vi "Merge Results.vi"(8 "error in (no error)":errorcluster, 9 "Merge in  front":bool, 10 "Result in":refnum<class "Acquired Result.lvclass">, 11 "Response Synchronizer in":refnum<class "Response Synchronizer.lvclass">) -> (0 "error out":errorcluster, 2 "Merged Result":refnum<class "Acquired Result.lvclass">, 3 "Response Synchronizer out":refnum<class "Response Synchronizer.lvclass">)   [LabVIEW 2021, in "Response Synchronizer.lvclass"]
uses:
  Response Synchronizer.lvclass
  NHMFL_Core/Libraries/Instruments/Results/Acquired Result/Acquired Result.lvclass
  Response Synchronizer.lvclass/Response Synchronizer.ctl
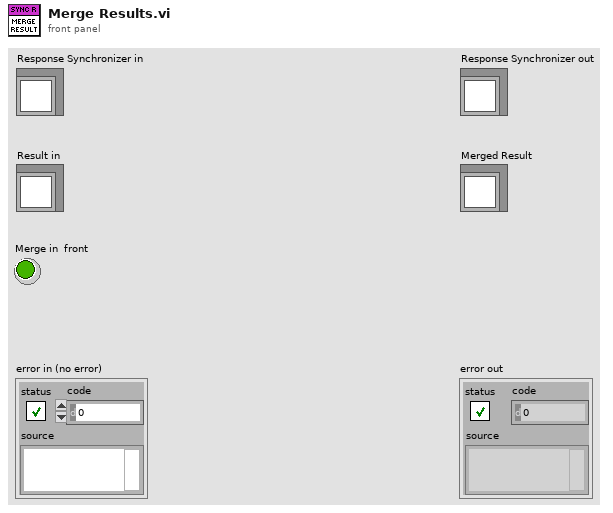
[diagram p1: front panel]
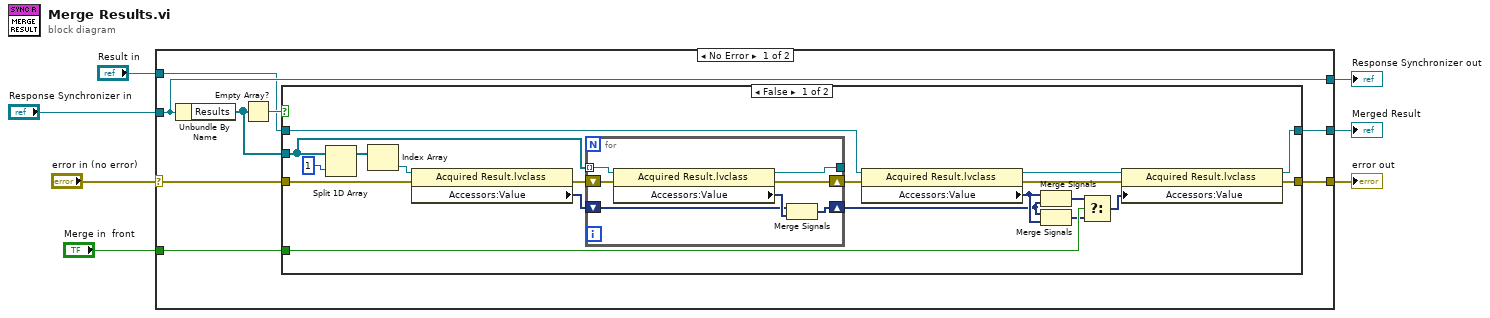
[diagram p0: block diagram]
diagram:
  n1 = case shown="No Error" "error in (no error)" {
    selector: "error in (no error)" -> [w9 w46]
    tunnel: [w8 w46] -> w6
    tunnel: [w15 w45] -> w4
    tunnel: "Response Synchronizer in" -> [w15 w45]
    tunnel: [w12 w44] -> w3
    tunnel: "Result in" -> [w11 w44]
    tunnel: "Merge in  front" -> [w10 _]
    frame No Error {
      n2 = Unbundle By Name(w15) -> ("Results"=w14:refnum<class "Acquired Result.lvclass">[])
      n3 = Empty Array?(array=w14) -> (empty?=w13:bool)
      n4 = case shown="False" w13 {
        tunnel: w14 -> [w33 _]
        tunnel: [w16 w43] -> w12
        tunnel: w11 -> [w27 w43]
        tunnel: w9 -> [w32 w42]
        tunnel: w10 -> [w26 _]
        tunnel: [w17 w42] -> w8
        frame False {
          n5 = Split 1D Array(array=w33, index=1) -> (first subarray=w31:refnum<class "Acquired Result.lvclass">[])  [unwired: 1 out]
          n6 = Index Array(array=w31) -> (element=w30:refnum<class "Acquired Result.lvclass">)  [unwired: 1 in]
          n7 = property class="Acquired Result.lvclass"(reference=w30, error in=w32) -> (error out=w29:errorcluster, "Accessors:Value"=w28:dynamicdata)  [unwired: 1 out]
          n8 = for {
            tunnel: w33 -> [w41] mode=indexing
            tunnel: [w40] -> _
            shift-right: [w37] -> w23
            shift-left: w28 -> [w36]
            shift-right: [w35] -> w21
            shift-left: w29 -> [w39]
            n9 = property class="Acquired Result.lvclass"(reference=w41, error in=w39) -> (reference out=w40:refnum<class "Acquired Result.lvclass">, error out=w35:errorcluster, "Accessors:Value"=w38:dynamicdata)
            n10 = Merge Signals(w36, w38) -> (w37:dynamicdata)
          }
          n11 = property class="Acquired Result.lvclass"(reference=w27, error in=w21) -> (reference out=w19:refnum<class "Acquired Result.lvclass">, error out=w18:errorcluster, "Accessors:Value"=w24:dynamicdata)
          n12 = Merge Signals(w24, w23) -> (w25:dynamicdata)
          n13 = Merge Signals(w23, w24) -> (w22:dynamicdata)
          n14 = Select(t=w25, s=w26, f=w22) -> (s? t:f=w20:dynamicdata)
          n15 = property class="Acquired Result.lvclass"(reference=w19, error in=w18, "Accessors:Value"=w20) -> (reference out=w16:refnum<class "Acquired Result.lvclass">, error out=w17:errorcluster)
        }
        frame True {
        }
      }
    }
    frame Error {
    }
  }
  "error out" <- w6
  "Response Synchronizer out" <- w4
  "Merged Result" <- w3
